vi "Value Strings.vi"(8 "error in (no error)":errorcluster, 11 "Group in":refnum<class "Group DBL.lvclass">) -> (0 "error out":errorcluster, 1 "Timestamps":dbl[](array[numeric]), 2 "Value Strings":string[](array[string]), 3 "Group out":refnum<class "Group DBL.lvclass">)   [LabVIEW 2020, in "Vecto.lvlib" / "Group DBL.lvclass"]
uses:
  Group DBL.lvclass
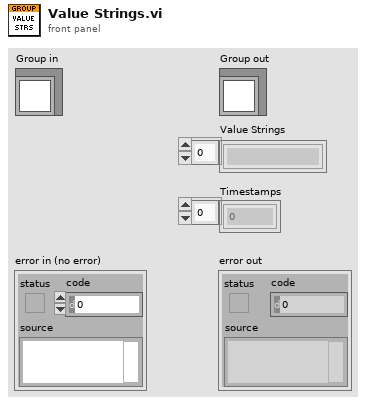
[diagram p1: front panel]
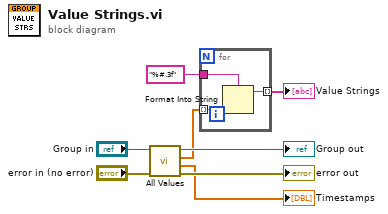
[diagram p0: block diagram]
diagram:
  n1 = call "All Values.vi"("error in (no error)"="error in (no error)", "Group in"="Group in") -> ("error out"=→"error out":errorcluster, "Timestamp"=→"Timestamps":dbl[], "Scaled"=w3:dbl[], "Group out"=→"Group out":refnum<class "Group DBL.lvclass">)  [unwired: 5 in, 1 out]
  n2 = for {
    tunnel: w3 -> [w11] mode=indexing
    tunnel: "%#.3f" -> [w10]
    tunnel: [w9] -> w1 mode=indexing
    n3 = Format Into String(format string=w10, w11) -> (resulting string=w9:string)  [unwired: 2 in, 1 out]
  }
  "Value Strings" <- w1
